vi "SS_CreateFileName.vi"(6 "Main Cluster IN":T1, 8 "Error In":errorcluster, 11 "Info In":string="\nWaiting for TimerScope Trigger\n- IN: SS TimerScope Trigger\n- OUT: SET SS ThermoRec Received Trigger\nPulse Number is 231123\nPulse Type is 4\n\nDuration (s) is  2.000000\nDelay (s)  is  1.000000\nScan Period (ms) is  15\nNumber of Samples is  134\n\nDelay Started\nDelay Complete\nExternal Measurement of Delay (s): 1.000000\nACQUIRING DATA") -> (0 "Error Out":errorcluster, 3 "Info Out":string="\nWaiting for TimerScope Trigger\n- IN: SS TimerScope Trigger\n- OUT: SET SS ThermoRec Received Trigger\nPulse Number is 231123\nPulse Type is 4\n\nDuration (s) is  2.000000\nDelay (s)  is  1.000000\nScan Period (ms) is  15\nNumber of Samples is  134\n\nDelay Started\nDelay Complete\nExternal Measurement of Delay (s): 1.000000\nACQUIRING DATA", 4 "Main Cluster OUT":T1)   [LabVIEW 2016]
uses:
  Control/Control_Main.ctl
  Control/Control_ModuleArray.ctl
panel:
  in  "Tab Control":enum32{"IN", "OUT", "SubVI Info"}(tab)
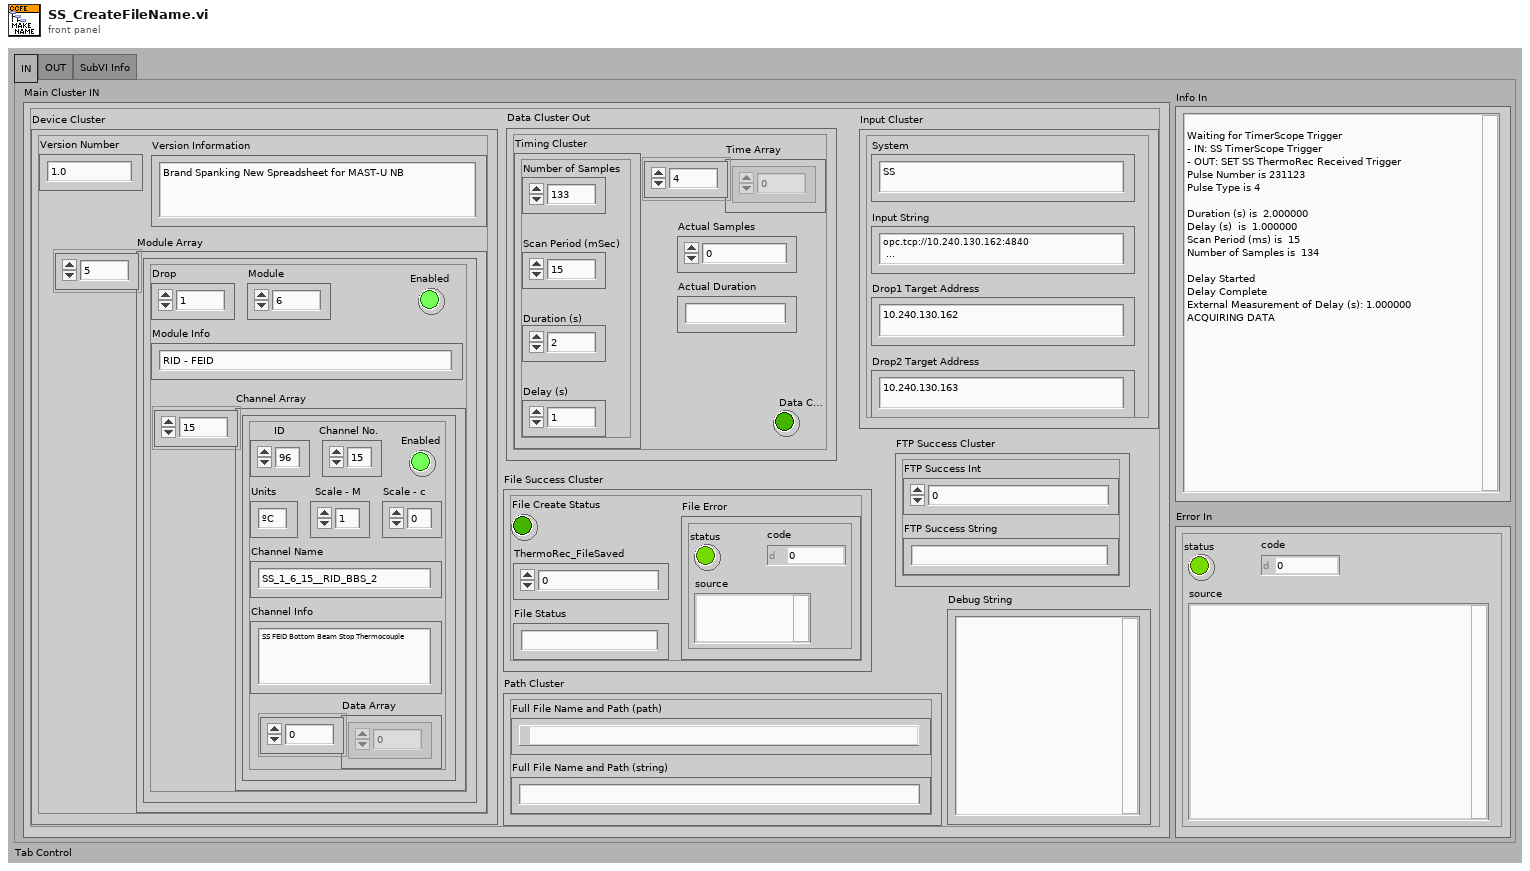
[diagram p1: front panel]
types:
  T1 = typedef "Control_Main.ctl" = cluster{"Device Cluster":cluster{"Module Array":T2, "Version Number":string, "Version Information":string}, "Input Cluster":cluster{"Input String":string, "Drop1 Target Address":string, "Drop2 Target Address":string, "System":string}, "Data Cluster Out":cluster{"Timing Cluster":cluster{"Number of Samples":i32, "Scan Period (mSec)":u32, "Duration (s)":dbl, "Delay (s)":dbl}, "Time Array":dbl[], "Actual Samples":i32, "Actual Duration":string, "Data Collection Error":bool}, "Path Cluster":cluster{"Full File Name and Path (path)":path, "Full File Name and Path (string)":string}, "File Success Cluster":cluster{"ThermoRec_FileSaved":i32, "File Create Status":bool, "File Error":errorcluster, "File Status":string}, "FTP Success Cluster":cluster{"FTP Success Int":i32, "FTP Success String":string}, "Debug String":string}
  T2 = typedef "Control_ModuleArray.ctl" = cluster{"Drop":i32, "Module":i32, "Module Info":string, "Enabled":bool, "Channel Array":cluster{"ID":i32, "Channel No.":i32, "Enabled":bool, "Channel Name":string, "Channel Info":string, "Units":string, "Scale - M":dbl, "Scale - c":dbl, "Data Array":dbl[]}[]}[]
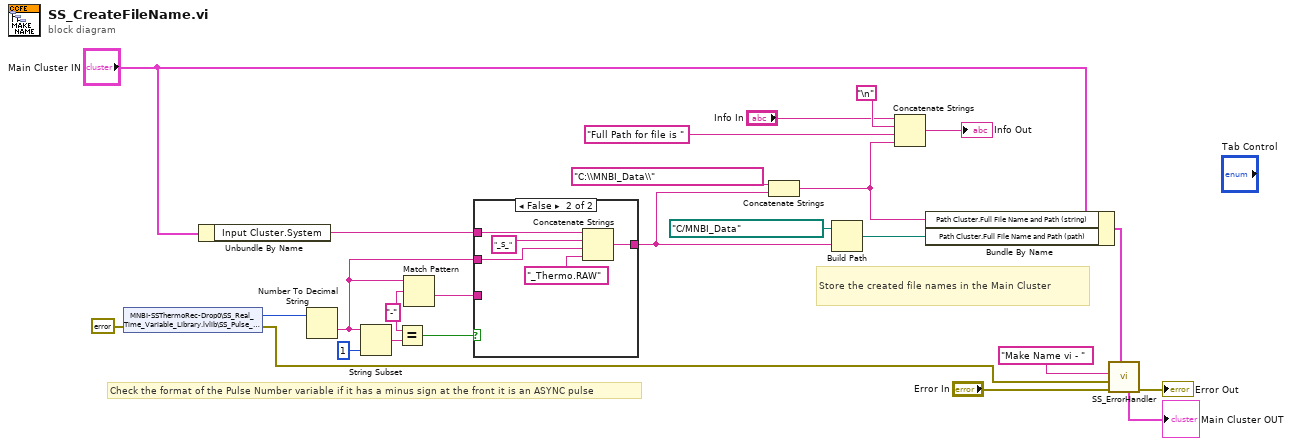
[diagram p0: block diagram]
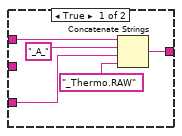
[diagram p2: hidden frame]
diagram:
  w21 = "-" ("y")
  # "Store the created file names in the Main Cluster"
  # "Check the format of the Pulse Number variable if it has a minus sign at the front it is an ASYNC pulse"
  n1 = shared-variable "MNBI-SSThermoRec-Drop0\\SS_Real_Time_Variable_Library.lvlib\\SS_Pulse_Number"(error in=errorcluster {"status"=FALSE, "code"=0, "source"=""} ("error in (no error)")) -> (w12:i32, error out=w1:errorcluster)
  n2 = Unbundle By Name("Main Cluster IN") -> ("Input Cluster.System"=w11:string)
  n3 = Number To Decimal String(number=w12) -> (decimal integer string=w24:string)  [unwired: 1 in]
  n4 = String Subset(string=w24, length (rest)=1 ("length (rest)")) -> (substring=w22:string)  [unwired: 1 in]
  n5 = Equal?(x=w21, y=w22) -> (x = y?=w23:bool)
  n6 = Match Pattern(string=w24, regular expression=w21) -> (after substring=w25:string)  [unwired: 1 in, 3 out]
  n7 = case shown="False" w23 {
    tunnel: w24 -> [_ w32]
    tunnel: w25 -> [w28 _]
    tunnel: w11 -> [w30 w35]
    tunnel: [w26 w31] -> w16
    frame True {
      n8 = Concatenate Strings(w30, "_A_", w28, "_Thermo.RAW") -> (w26:string)
    }
    frame False {
      n9 = Concatenate Strings(w35, "_S_", w32, "_Thermo.RAW") -> (w31:string)
    }
  }
  n10 = Concatenate Strings("C:\\MNBI_Data\\", w16) -> (w15:string)
  n11 = Build Path(base path=path "C:/MNBI_Data" ("path"), name or relative path=w16) -> (appended path=w18:path)
  n12 = Concatenate Strings("Info In", "\n", "Full Path for file is ", w15) -> (→"Info Out":string)
  n13 = Bundle By Name(cluster="Main Cluster IN", "Path Cluster.Full File Name and Path (string)"=w15, "Path Cluster.Full File Name and Path (path)"=w18) -> (w3:T1)
  n14 = call "SS_ErrorHandler.vi"("Main Cluster IN"=w3, "Error In"="Error In", "SubVI Error"=w1, "SubVI Name"="Make Name vi - ") -> ("Error Out"=→"Error Out":errorcluster, "Main Cluster OUT"=→"Main Cluster OUT":T1)  [unwired: 5 in, 1 out]
